vi "ADI_IMU_ADIS16448_FGV.vi"(0 "ADI IMU DevRef":T1={"DevStatus"={"status"=FALSE, "code"=0, "source"=""}, "Handle"=0, "SPI Bus"=enum."SPI On-Board, CS0", "Device Found"=FALSE, "Device Ready"=FALSE, "Yaw Axis"=enum."Z", "AHRS Algorithm"=enum."Complementary", "Serial"=0, "Lot ID 2"=0, "Lot ID 1"=0, "Bytes Per Sample"=0, "Calibrate On Open?"=FALSE}, 1 "Operation":enum16{"set", "get", "set reset"}(ring), 2 "Sensor Ready?":bool, 5 "Reset":bool, 7 "IMU Data":T5, 9 "IMU Angles":T3, 11 "IMU AHRS":cluster{"Pitch":dbl, "Roll":dbl, "Yaw":dbl}, 12 "Offset Compensated Data":dbl[](array[numeric])) -> (4 "ADI IMU DevRef Out":T1={"DevStatus"={"status"=FALSE, "code"=0, "source"=""}, "Handle"=0, "SPI Bus"=enum."SPI On-Board, CS0", "Device Found"=FALSE, "Device Ready"=FALSE, "Yaw Axis"=enum."Z", "AHRS Algorithm"=enum."Complementary", "Serial"=0, "Lot ID 2"=0, "Lot ID 1"=0, "Bytes Per Sample"=0, "Calibrate On Open?"=FALSE}, 6 "Reset Out":bool, 8 "IMU Data Out":T4, 10 "IMU Angles Out":T3, 13 "Sensor Ready Out":bool, 14 "Offset Compensated Data Out":dbl[](array[numeric]), 15 "IMU AHRS Out":cluster{"Pitch":dbl, "Roll":dbl, "Yaw":dbl})   [LabVIEW 2018, in "ADIS16448_IMU.lvlib"]
uses:
  ADIS16448_IMU.lvlib
  ADI_IMU_ADIS16448_IMUDevRef.ctl
  <vilib>/Rock Robotics/SystemInterfaces/spilib/spi_bus.ctl
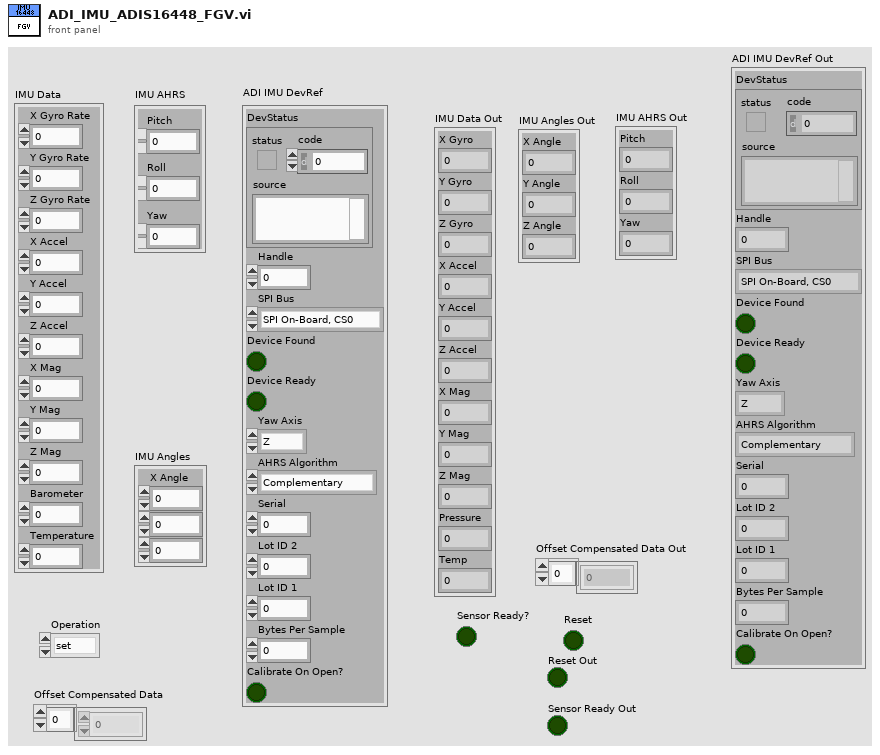
[diagram p1: front panel]
types:
  T1 = typedef "ADIS16448_IMU.lvlib/ADI_IMU_ADIS16448_IMUDevRef.ctl" = cluster{"DevStatus":errorcluster, "Handle":i32, "SPI Bus":T2, "Device Found":bool, "Device Ready":bool, "Yaw Axis":enum16{"X", "Y", "Z"}, "AHRS Algorithm":enum16{"Complementary", "Madgwick"}, "Serial":u16, "Lot ID 2":u16, "Lot ID 1":u16, "Bytes Per Sample":u16, "Calibrate On Open?":bool}
  T2 = typedef "spi_bus.ctl" = enum16{"SPI On-Board, CS0", "SPI On-Board, CS1", "SPI On-Board, CS2", "SPI On-Board, CS3", "SPI MXP", "Invalid"}
  T3 = cluster{"X Angle":dbl, "Y Angle":dbl, "Z Angle":dbl}
  T4 = cluster{"X Gyro":dbl, "Y Gyro":dbl, "Z Gyro":dbl, "X Accel":dbl, "Y Accel":dbl, "Z Accel":dbl, "X Mag":dbl, "Y Mag":dbl, "Z Mag":dbl, "Pressure":dbl, "Temp":dbl}
  T5 = cluster{"X Gyro Rate":dbl, "Y Gyro Rate":dbl, "Z Gyro Rate":dbl, "X Accel":dbl, "Y Accel":dbl, "Z Accel":dbl, "X Mag":dbl, "Y Mag":dbl, "Z Mag":dbl, "Barometer":dbl, "Temperature":dbl}
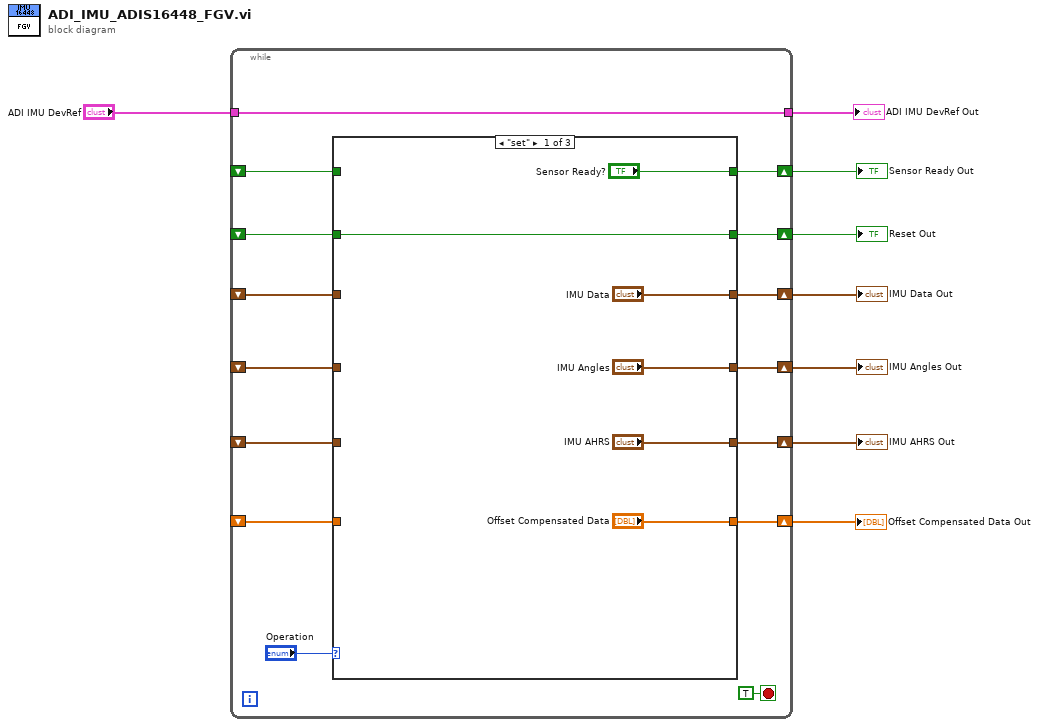
[diagram p0: block diagram]
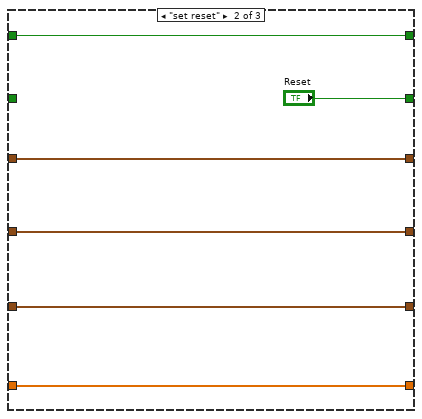
[diagram p2: hidden frame]
diagram:
  n1 = while {
    shift-right: [w21] -> w8
    shift-left: _ -> [w15]
    shift-right: [w20] -> w5
    shift-left: _ -> [w16]
    tunnel: "ADI IMU DevRef" -> [w19]
    tunnel: [w19] -> w6
    shift-right: [w18] -> w4
    shift-left: _ -> [w17]
    shift-right: [w14] -> w3
    shift-left: _ -> [w13]
    shift-right: [w12] -> w1
    shift-left: _ -> [w11]
    shift-right: [w9] -> w7
    shift-left: _ -> [w10]
    stop <- TRUE stop-if-true
    n2 = case shown="\"set\"" "Operation" {
      tunnel: [w25 "Reset" w39] -> w21
      tunnel: ["IMU Data" w31 w40] -> w20
      tunnel: ["IMU Angles" w32 w41] -> w18
      tunnel: w17 -> [_ w32 w41]
      tunnel: w16 -> [_ w31 w40]
      tunnel: w15 -> [w25 _ w39]
      tunnel: ["IMU AHRS" w33 w38] -> w14
      tunnel: w13 -> [_ w33 w38]
      tunnel: ["Offset Compensated Data" w34 w37] -> w12
      tunnel: w11 -> [_ w34 w37]
      tunnel: ["Sensor Ready?" w30 w36] -> w9
      tunnel: w10 -> [_ w30 w36]
      frame "set" {
      }
      frame "set reset" {
      }
      frame "get", Default {
      }
    }
  }
  "Reset Out" <- w8
  "Sensor Ready Out" <- w7
  "IMU Data Out" <- w5
  "IMU Angles Out" <- w4
  "IMU AHRS Out" <- w3
  "ADI IMU DevRef Out" <- w6
  "Offset Compensated Data Out" <- w1
